vi "ESA-C Voltage To Position.vi"(1 "Axis":i32, 2 "Voltage (V)":dbl) -> (0 "Position (µm)":dbl)   [LabVIEW 2010]
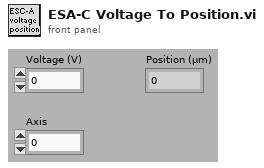
[diagram p1: front panel]
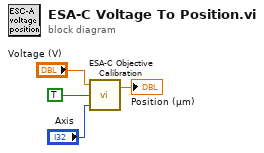
[diagram p0: block diagram]
diagram:
  n1 = call "ESA-C Objective Calibration.vi"("Axis"="Axis", "Is Voltage?"=TRUE, "Input Value"="Voltage (V)") -> ("Output Value"=→"Position (µm)":dbl)  [unwired: 1 in]
